vi "LeerBD.vi"(8 "error in (no error)":errorcluster) -> (0 "error out":errorcluster, 2 "BD":T1={"frec_referencia"=98.0, "niv_presion_son_ref"=97.0, "RangoMaxRef(dB)"=98.0, "Incertidumbre"=["1", "1", "1", "1", "1", "1", "1", "1", "1", "1"], "Tol +"=["2,0", "1,5", "1,5", "1,4", "1,4", "1,1", "1,6", "1,6", "2,1", "3,5"], "Tol -"=["-2,0", "-1,5", "-1,5", "-1,4", "-1,4", "-1,1", "-1,6", "-1,6", "-2,1", "-3,5"], "Frecuencias(Hz)"=["95", "94", "94", "94", "96", "95", "94", "96", "95", "94"], "vol_enviado_CAM"=0.0, "Ponderaciones A"=[0.0, 0.0, 0.0, 0.0, 0.0, 0.0, 0.0, 0.0, 0.0, 0.0], "Ponderaciones C"=[0.0, 0.0, 0.0, 0.0, 0.0, 0.0, 0.0, 0.0, 0.0, 0.0], "Ponderaciones Z"=[0.0, 0.0, 0.0, 0.0, 0.0, 0.0, 0.0, 0.0, 0.0, 0.0]}, 3 "Prueba04 out":refnum<class "Prueba04.lvclass">)   [LabVIEW 2019, in "Prueba04.lvclass"]
uses:
  Prueba04.lvclass
  Control/BD.ctl
  Base de Datos/SQLiteConnector/SQLiteConnection.lvclass
  Base de Datos/Base de Datos.lvclass
panel:
  in  "Tipo Equipo":enum16{"Sonometro", "Calibrador", "Dosimetro"}(ring)
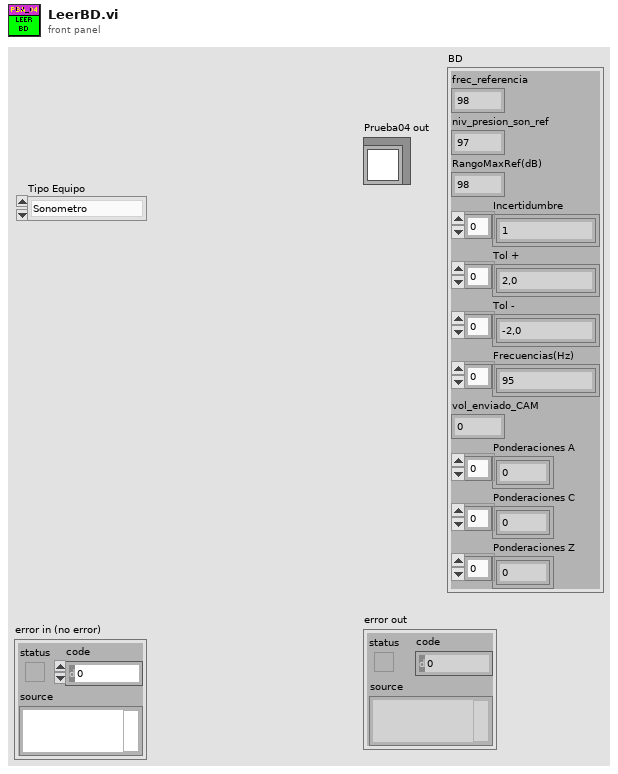
[diagram p1: front panel]
types:
  T1 = typedef "Prueba04.lvclass/BD.ctl" = cluster{"frec_referencia":dbl, "niv_presion_son_ref":dbl, "RangoMaxRef(dB)":dbl, "Incertidumbre":string[], "Tol +":string[], "Tol -":string[], "Frecuencias(Hz)":string[], "vol_enviado_CAM":dbl, "Ponderaciones A":dbl[], "Ponderaciones C":dbl[], "Ponderaciones Z":dbl[]}
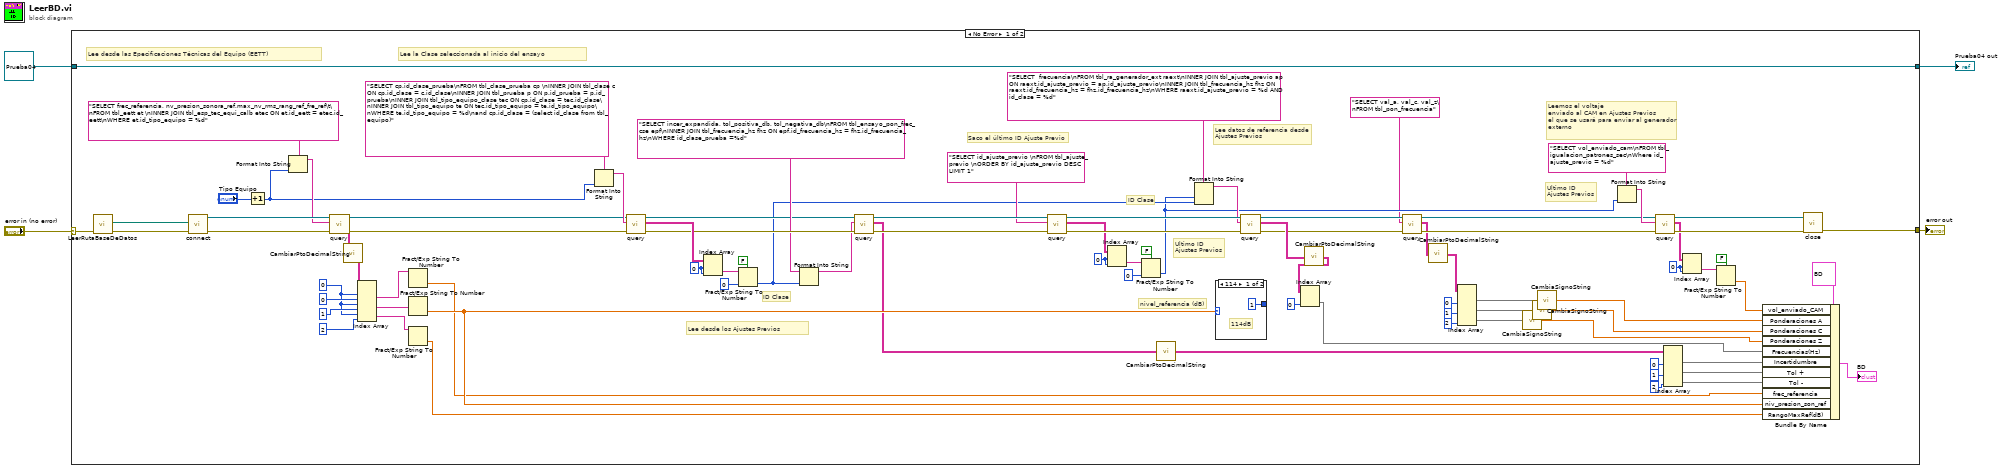
[diagram p0: block diagram]
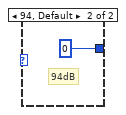
[diagram p2: hidden frame]
diagram:
  n1 = case shown="No Error" "error in (no error)" {
    selector: "error in (no error)" -> [w85 w97]
    tunnel: [w69 w97] -> w3
    tunnel: [w93 w96] -> w1
    tunnel: refnum<class "Prueba04.lvclass"> refnum ("Prueba02 in") -> [w93 w96]
    frame No Error {
      w33 = 0 ("index (row)")
      w47 = 0 ("index (row)")
      w75 = 0 ("index (row)")
      w31 = 0 ("index (row)")
      # "Ultimo ID\nAjustes Previos"
      # "Ultimo ID\nAjustes Previos"
      # "ID Clase"
      # "Leemos el voltaje\nenviado al CAM en Ajustes Previos\nel que se usará para enviar al generador\nexterno"
      # "Lee datos de referencia desde\nAjustes Previos"
      # "ID Clase"
      # "Saco el último ID Ajuste Previo"
      # "nivel_referencia (dB)"
      # "Lee desde los Ajustes Previos"
      # "Lee la Clase seleccionada al inicio del ensayo"
      # "Lee desde las Epecificaciones Técnicas del Equipo (EETT)"
      n2 = call "LeerRutaBaseDeDatos.vi"("error in (no error)"=w85) -> ("error out"=w88:errorcluster, "Database Path"=w87:path)  [unwired: 9 in]
      n3 = call "connect.vi"("error in (no error)"=w88, "Database Path"=w87) -> ("error out"=w90:errorcluster, "object out"=w91:refnum<class "SQLiteConnection.lvclass">)  [unwired: 8 in]
      n4 = Increment(x="Tipo Equipo") -> (x+1=w64:enum16{"Sonometro", "Calibrador", "Dosimetro"})
      n5 = Format Into String(format string="SELECT frec_referencia, nv_presion_sonora_ref,max_nv_rms_rang_ref_fre_ref\t\nFROM tbl_eett et \nINNER JOIN tbl_esp_tec_equi_calb etec ON et.id_eett = etec.id_eett\nWHERE et.id_tipo_equipo = %d", w64) -> (resulting string=w89:string)  [unwired: 2 in, 1 out]
      n6 = call "query.vi"("error in (no error)"=w90, "SQL Statement"=w89, "object in"=w91) -> ("error out"=w76:errorcluster, "result"=w80:string[][], "object out"=w77:refnum<class "SQLiteConnection.lvclass">)  [unwired: 5 in, 1 out]
      n7 = call "CambiarPtoDecimalString.vi"("result"=w80) -> ("result out"=w22:string[][])
      n8 = Index Array(array=w22, index (row) #1=w31, index (col) #1=0 ("disabled index (col)"), index (row) #2=w31, index (col) #2=1 ("disabled index (col)"), index (row) #3=w31, index (col) #3=2 ("disabled index (col)")) -> (element #1=w82:string, element #2=w81:string, element #3=w29:string)
      n9 = Fract/Exp String To Number(string=w82) -> (number=w55:dbl)  [unwired: 3 in, 1 out]
      n10 = Fract/Exp String To Number(string=w81) -> (number=w63:dbl)  [unwired: 3 in, 1 out]
      n11 = Fract/Exp String To Number(string=w29) -> (number=w26:dbl)  [unwired: 3 in, 1 out]
      n12 = Format Into String(format string="SELECT cp.id_clase_prueba\nFROM tbl_clase_prueba cp \nINNER JOIN tbl_clase c ON cp.id_clase = c.id_clase\nINNER JOIN tbl_prueba p ON p.id_prueba = p.id_prueba\nINNER JOIN tbl_tipo_equipo_clase tec ON cp.id_clase = tec.id_clase\nINNER JOIN tbl_tipo_equipo te ON tec.id_tipo_equipo = te.id_tipo_equipo\nWHERE te.id_tipo_equipo = %d\nand cp.id_clase = (select id_clase from tbl_equipo)", w64) -> (resulting string=w78:string)  [unwired: 2 in, 1 out]
      n13 = call "query.vi"("error in (no error)"=w76, "SQL Statement"=w78, "object in"=w77) -> ("error out"=w70:errorcluster, "result"=w71:string[][], "object out"=w66:refnum<class "SQLiteConnection.lvclass">)  [unwired: 5 in, 1 out]
      n14 = Index Array(array=w71, index (row)=w75, index (col)=w75) -> (element=w73:string)
      n15 = Fract/Exp String To Number(use system decimal point (T)=FALSE, string=w73, default (0 dbl)=0 ("index (row)")) -> (number=w43:i32)  [unwired: 1 in, 1 out]
      n16 = Format Into String(format string="SELECT incer_expandida, tol_positiva_db, tol_negativa_db\nFROM tbl_ensayo_pon_frec_cse epf\nINNER JOIN tbl_frecuencia_hz fhz ON epf.id_frecuencia_hz = fhz.id_frecuencia_hz\nWHERE id_clase_prueba =%d", w43) -> (resulting string=w65:string)  [unwired: 2 in, 1 out]
      n17 = call "query.vi"("error in (no error)"=w70, "SQL Statement"=w65, "object in"=w66) -> ("error out"=w67:errorcluster, "result"=w59:string[][], "object out"=w53:refnum<class "SQLiteConnection.lvclass">)  [unwired: 5 in, 1 out]
      n18 = call "query.vi"("error in (no error)"=w67, "SQL Statement"="SELECT id_ajuste_previo \nFROM tbl_ajuste_previo \nORDER BY id_ajuste_previo DESC LIMIT 1" ("format string"), "object in"=w53) -> ("error out"=w54:errorcluster, "result"=w46:string[][], "object out"=w52:refnum<class "SQLiteConnection.lvclass">)  [unwired: 5 in, 1 out]
      n19 = Index Array(array=w46, index (row)=w47, index (col)=w47) -> (element=w49:string)
      n20 = Fract/Exp String To Number(use system decimal point (T)=FALSE, string=w49, default (0 dbl)=0 ("index (row)")) -> (number=w36:i32)  [unwired: 1 in, 1 out]
      n21 = call "CambiarPtoDecimalString.vi"("result"=w59) -> ("result out"=w23:string[][])
      n22 = Format Into String(format string="SELECT  frecuencia\nFROM tbl_ra_generador_ext raext\nINNER JOIN tbl_ajuste_previo ap ON raext.id_ajuste_previo = ap.id_ajuste_previo\nINNER JOIN tbl_frecuencia_hz fhz ON raext.id_frecuencia_hz = fhz.id_frecuencia_hz\nWHERE raext.id_ajuste_previo = %d AND id_clase = %d", w36, w43) -> (resulting string=w44:string)  [unwired: 2 in, 1 out]
      n23 = case shown="114" w63 {
        tunnel: [1 ("disabled index (col)") 0 ("disabled index (col)")] -> _
        frame 114 {
          # "114dB"
        }
        frame 94, Default {
          # "94dB"
        }
      }
      n24 = call "query.vi"("error in (no error)"=w54, "SQL Statement"=w44, "object in"=w52) -> ("error out"=w19:errorcluster, "result"=w25:string[][], "object out"=w21:refnum<class "SQLiteConnection.lvclass">)  [unwired: 5 in, 1 out]
      n25 = call "CambiarPtoDecimalString.vi"("result"=w25) -> ("result out"=w24:string[][])
      n26 = Index Array(array=w24, index (col)=0 ("disabled index (col)")) -> (element=w41:string[])  [unwired: 1 in]
      n27 = call "query.vi"("error in (no error)"=w19, "SQL Statement"="SELECT val_a, val_c, val_z\nFROM tbl_pon_frecuencia" ("format string"), "object in"=w21) -> ("error out"=w18:errorcluster, "result"=w15:string[][], "object out"=w20:refnum<class "SQLiteConnection.lvclass">)  [unwired: 5 in, 1 out]
      n28 = call "CambiarPtoDecimalString.vi"("result"=w15) -> ("result out"=w14:string[][])
      n29 = Index Array(array=w14, index (col) #1=0 ("disabled index (col)"), index (col) #2=1 ("index (col)"), index (col) #3=2 ("index (col)")) -> (element #1=w10:string[], element #2=w9:string[], element #3=w8:string[])  [unwired: 3 in]
      n30 = call "CambiaSignoString.vi"("result"=w8) -> ("result out"=w5:dbl[])
      n31 = call "CambiaSignoString.vi"("result"=w9) -> ("result out"=w6:dbl[])
      n32 = call "CambiaSignoString.vi"("result"=w10) -> ("result out"=w7:dbl[])
      n33 = Format Into String(format string="SELECT vol_enviado_cam\nFROM tbl_igualacion_patrones_sec\nWhere id_ajuste_previo = %d", w36) -> (resulting string=w37:string)  [unwired: 2 in, 1 out]
      n34 = call "query.vi"("error in (no error)"=w18, "SQL Statement"=w37, "object in"=w20) -> ("error out"=w40:errorcluster, "result"=w32:string[][], "object out"=w39:refnum<class "SQLiteConnection.lvclass">)  [unwired: 5 in, 1 out]
      n35 = Index Array(array=w23, index (col) #1=0 ("disabled index (col)"), index (col) #2=1 ("index (col)"), index (col) #3=2 ("index (col)")) -> (element #1=w62:string[], element #2=w61:string[], element #3=w60:string[])  [unwired: 3 in]
      n36 = Index Array(array=w32, index (row)=w33, index (col)=w33) -> (element=w35:string)
      n37 = Fract/Exp String To Number(use system decimal point (T)=FALSE, string=w35) -> (number=w13:dbl)  [unwired: 2 in, 1 out]
      n38 = Bundle By Name(cluster=T1 {"frec_referencia"=98.0, "niv_presion_son_ref"=97.0, "RangoMaxRef(dB)"=98.0, "Incertidumbre"=["1", "1", "1", "1", "1", "1", "1", "1", "1", "1"], "Tol +"=["2,0", "1,5", "1,5", "1,4", "1,4", "1,1", "1,6", "1,6", "2,1", "3,5"], "Tol -"=["-2,0", "-1,5", "-1,5", "-1,4", "-1,4", "-1,1", "-1,6", "-1,6", "-2,1", "-3,5"], "Frecuencias(Hz)"=["95", "94", "94", "94", "96", "95", "94", "96", "95", "94"], "vol_enviado_CAM"=0.0, "Ponderaciones A"=[0.0, 0.0, 0.0, 0.0, 0.0, 0.0, 0.0, 0.0, 0.0, 0.0], "Ponderaciones C"=[0.0, 0.0, 0.0, 0.0, 0.0, 0.0, 0.0, 0.0, 0.0, 0.0], "Ponderaciones Z"=[0.0, 0.0, 0.0, 0.0, 0.0, 0.0, 0.0, 0.0, 0.0, 0.0]} ("BD"), "vol_enviado_CAM"=w13, "Ponderaciones A"=w7, "Ponderaciones C"=w6, "Ponderaciones Z"=w5, "Frecuencias(Hz)"=w41, "Incertidumbre"=w62, "Tol +"=w61, "Tol -"=w60, "frec_referencia"=w55, "niv_presion_son_ref"=w63, "RangoMaxRef(dB)"=w26) -> (→"BD":T1)
      n39 = call-dynamic "close.vi"("error in (no error)"=w40, "object in"=w39) -> ("error out"=w69:errorcluster)  [unwired: 8 in, 1 out]
    }
    frame Error {
    }
  }
  "error out" <- w3
  "Prueba04 out" <- w1
